vi "FastICA.vi"(8 "error in":errorcluster) -> (0 "error out":errorcluster, 3 "out":refnum<class "FastICA.lvclass">)   [LabVIEW 2020]
doc: "FastICA: a fast algorithm for Independent Component Analysis.\n\n Read more in the :ref:`User Guide <ICA>`.\n\n Parameters\n ----------\n n_components : int, default=None\n Number of components to use. If None is passed, all are used.\n\n algorithm : {'parallel', 'deflation'}, default='parallel'\n Apply parallel or deflational algorithm for FastICA.\n\n whiten : bool, default=True\n If whiten is false, the data is already considered to be\n whitened, and no whitening is performed.\n\n fun : {'logcosh', 'exp', 'cube'} or callable, default='logcosh'\n The functional form of the G function used in the\n approximation to neg-entropy. Could be either 'logcosh', 'exp',\n or 'cube'.\n You can also provide your own function. It should return a tuple\n containing the value of the function, and of its derivative, in the\n point. Example::\n\n def my_g(x):\n return x ** 3, (3 * x ** 2).mean(axis=-1)\n\n fun_args : dict, default=None\n Arguments to send to the functional form.\n If empty and if fun='logcosh', fun_args will take value\n {'alpha' : 1.0}.\n\n max_iter : int, default=200\n Maximum number of iterations during fit.\n\n tol : float, default=1e-4\n Tolerance on update at each iteration.\n\n w_init : ndarray of shape (n_components, n_components), default=None\n The mixing matrix to be used to initialize the algorithm.\n\n random_state : int, RandomState instance or None, default=None\n Used to initialize ``w_init`` when not specified, with a\n normal distribution. Pass an int, for reproducible results\n across multiple function calls.\n See :term:`Glossary <random_state>`.\n\n Attributes\n ----------\n components_ : ndarray of shape (n_components, n_features)\n The linear operator to apply to the data to get the independent\n sources. This is equal to the unmixing matrix when ``whiten`` is\n False, and equal to ``np.dot(unmixing_matrix, self.whitening_)`` when\n ``whiten`` is True.\n\n mixing_ : ndarray of shape (n_features, n_components)\n The pseudo-inverse of ``components_``. It is the linear operator\n that maps independent sources to the data.\n\n mean_ : ndarray of shape(n_features,)\n The mean over features. Only set if `self.whiten` is True.\n\n n_iter_ : int\n If the algorithm is \"deflation\", n_iter is the\n maximum number of iterations run across all components. Else\n they are just the number of iterations taken to converge.\n\n whitening_ : ndarray of shape (n_components, n_features)\n Only set if whiten is 'True'. This is the pre-whitening matrix\n that projects data onto the first `n_components` principal components.\n\n \nAvailable methods:\nFit\nFit Transform\nTransform\nGet Attributes\nGet Params\nSet Params"
uses:
  FastICA.lvclass
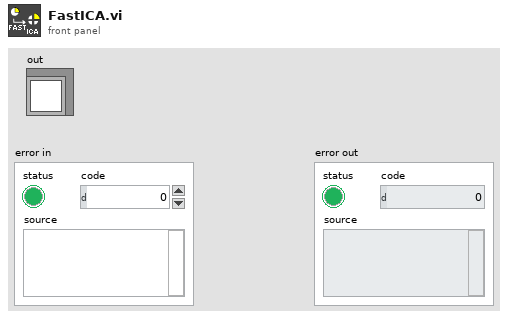
[diagram p1: front panel]
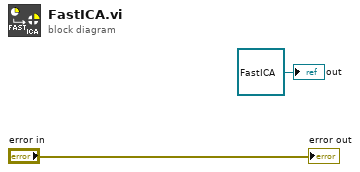
[diagram p0: block diagram]
diagram:
  "out" <- refnum<class "FastICA.lvclass"> refnum ("model")
  "error out" <- "error in"
